vi "8116-SpectraSaver.vi"(10 "base path":path, 11 "Ch3MeanSpec":dbl[](array[numeric])) -> ()   [LabVIEW 2016]
uses:
  EnFloSW/Anemometry/Anemometry Sub Vis/Globals/Meas_global.vi
  <vilib>/Utility/file.llb/Write Delimited Spreadsheet (string).vi
panel:
  out "appended array":string[](array[string])
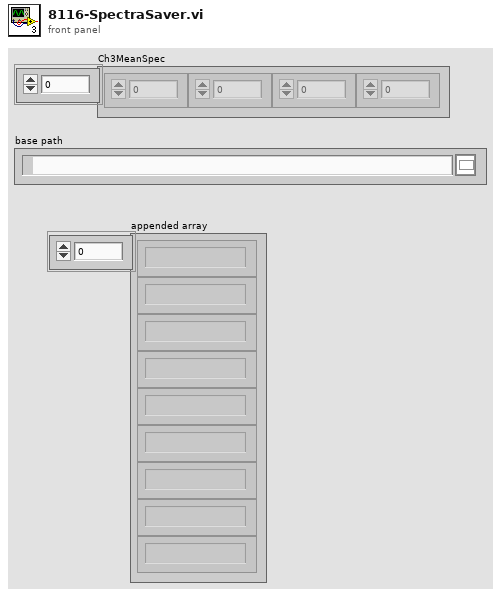
[diagram p1: front panel]
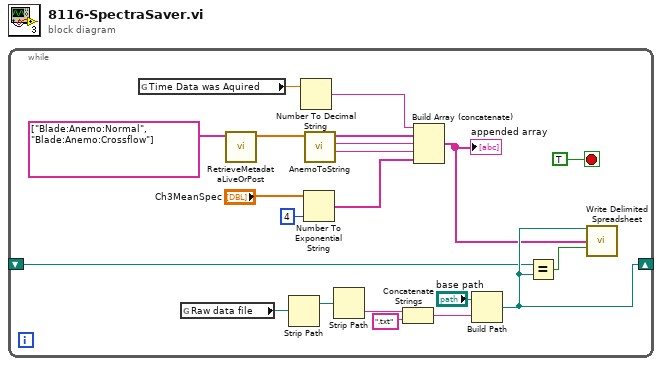
[diagram p0: block diagram]
diagram:
  n1 = while {
    shift-right: [w16] -> _
    shift-left: _ -> [w15]
    stop <- TRUE stop-if-true
    n2 = global read "Meas_global.vi" "Time Data was Aquired"() -> (w9:dbl)
    n3 = global read "Meas_global.vi" "Raw data file"() -> (w1:path)
    n4 = call "RetrieveMetadataLiveOrPost.vi"("Array in"=string[] ["Blade:Anemo:Normal", "Blade:Anemo:Crossflow"]) -> ("Array out"=w20:dbl[])  [unwired: 10 in]
    n5 = Strip Path(path=w1) -> (stripped path=w19:path)  [unwired: 1 out]
    n6 = Number To Decimal String(number=w9) -> (decimal integer string=w10:string)  [unwired: 1 in]
    n7 = Number To Exponential String(number="Ch3MeanSpec", precision (6)=i16 4) -> (E-format string=w3:string[])  [unwired: 2 in]
    n8 = call "AnemoToString.vi"("Normal,Crossflow"=w20) -> ("Theta"=w4:string, "Vmag"=w5:string, "Normal,Crossflow"=w6:string[])  [unwired: 8 in]
    n9 = Strip Path(path=w19) -> (name=w18:string)  [unwired: 1 out]
    n10 = Concatenate Strings(w18, ".txt" ("string")) -> (w13:string)
    n11 = Build Array (concatenate)(w10, w6, w5, w4, w3) -> (w2:string[])
    "appended array" <- w2
    n12 = Build Path(base path="base path", name or relative path=w13) -> (appended path=w16:path)
    n13 = Equal?(x=w15, y=w16) -> (x = y?=w17:bool)
    n14 = call-poly <vilib>:"Write Delimited Spreadsheet.vi"("file path (dialog if empty)"=w16, "1D data"=w2, "append to file? (new file:F)"=w17) -> ()  [unwired: 11 in, 2 out]
  }
